vi "base.vi"() -> ()   [LabVIEW 2017]
uses:
  <vilib>/Analysis/baseanly.llb/Inverse f Filter (DBL).vi
  <vilib>/Analysis/NI_AALBase.lvlib
panel:
  out "LED":bool
  in  "stop 3":bool
  in  "Amplitude du signal":dbl(knob) scale=0.0..10.0
  out "Valeur pic à pic du signal":dbl
  out "Graphe 2":dynamicdata(graph)
  in  "Bouton rotatif":dbl(knob) scale=0.0..10.0
  in  "stop 2":bool
  out "Graphe":dynamicdata(graph)
  out "Tableau aléatoire de nombres compris entre 0 et 20":dbl[](array[numeric])
  in  "stop":bool
  out "u":dbl[](array[numeric])
  in  "u0":dbl
  in  "q":dbl
  out "LED":bool
  in  "a":bool
  in  "b":bool
  in  "Numérique":i32
  out "u(n)":dbl[](array[numeric])
  out "u(N)":dbl
  in  "N":dbl
  out "sqrt(z)":dbl
  in  "z":dbl
  out "x = y ?":bool
  out "x < y ?":bool
  out "x > y ?":bool
  in  "Y":dbl
  in  "X":dbl
  out "F":dbl(slide) scale=0.0..100.0
  in  "C":dbl(slide) scale=0.0..100.0
  out "c 4":dbl
  in  "b 4":dbl
  in  "a 4":dbl
  out "c 3":dbl
  in  "b 3":dbl
  in  "a 3":dbl
  out "c 2":dbl
  in  "b 2":dbl
  in  "a 2":dbl
  out "c":dbl
  in  "b":dbl
  in  "a":dbl
  # "+"
  # "-"
  # "x"
  # "/"
  # "°F = 1,8 x °C + 32"
  # "u(N) = 2N + 1"
  # "u(n) = 3n+4"
  # "a ET b"
  # "suite géométrique"
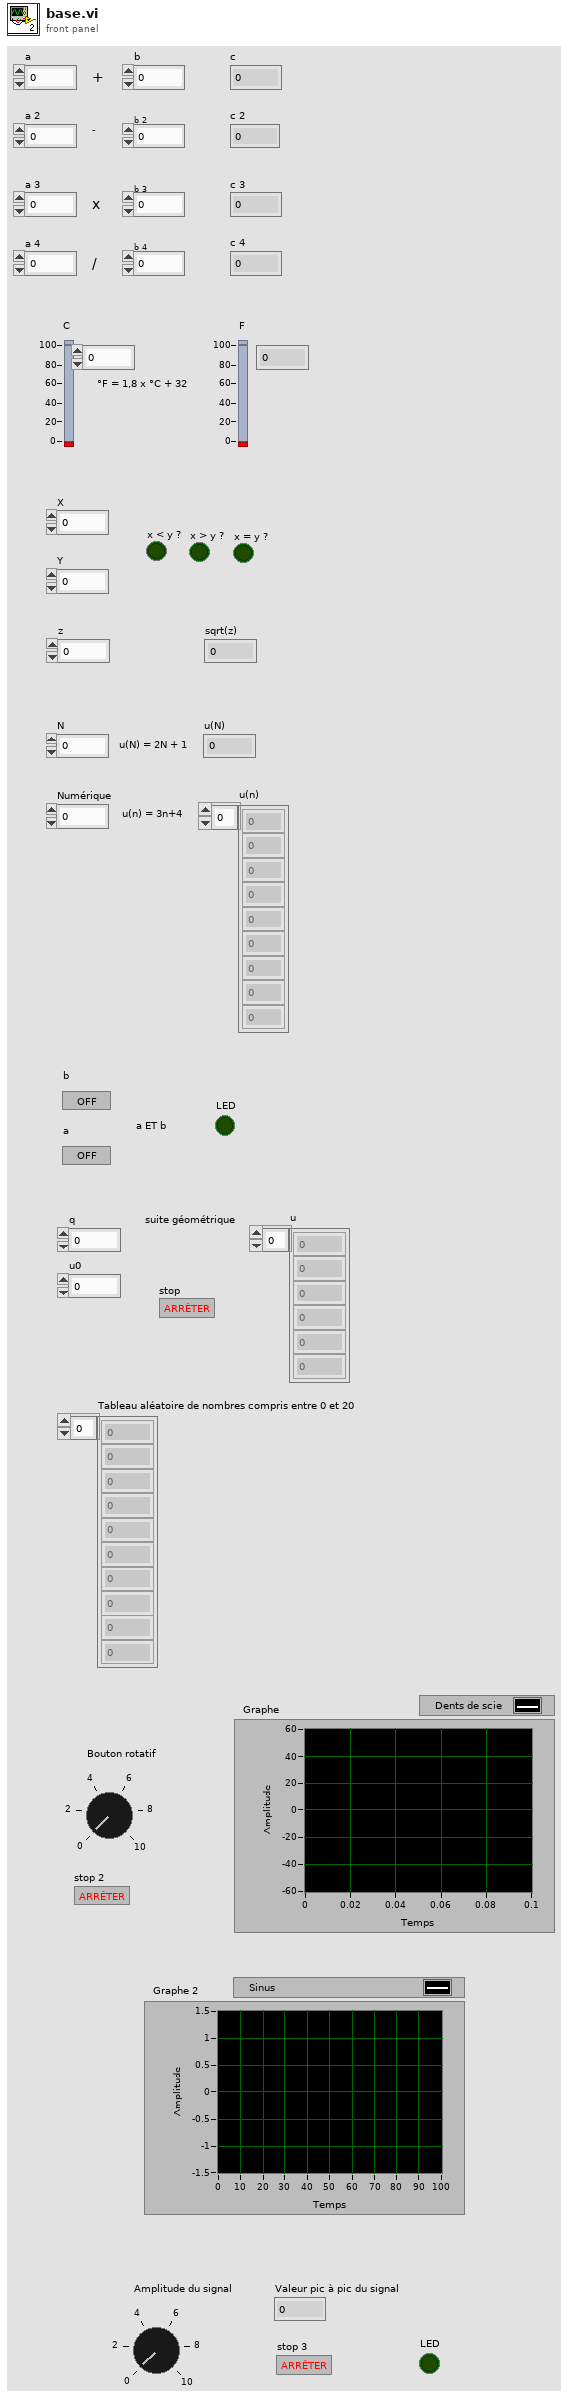
[diagram p1: front panel]
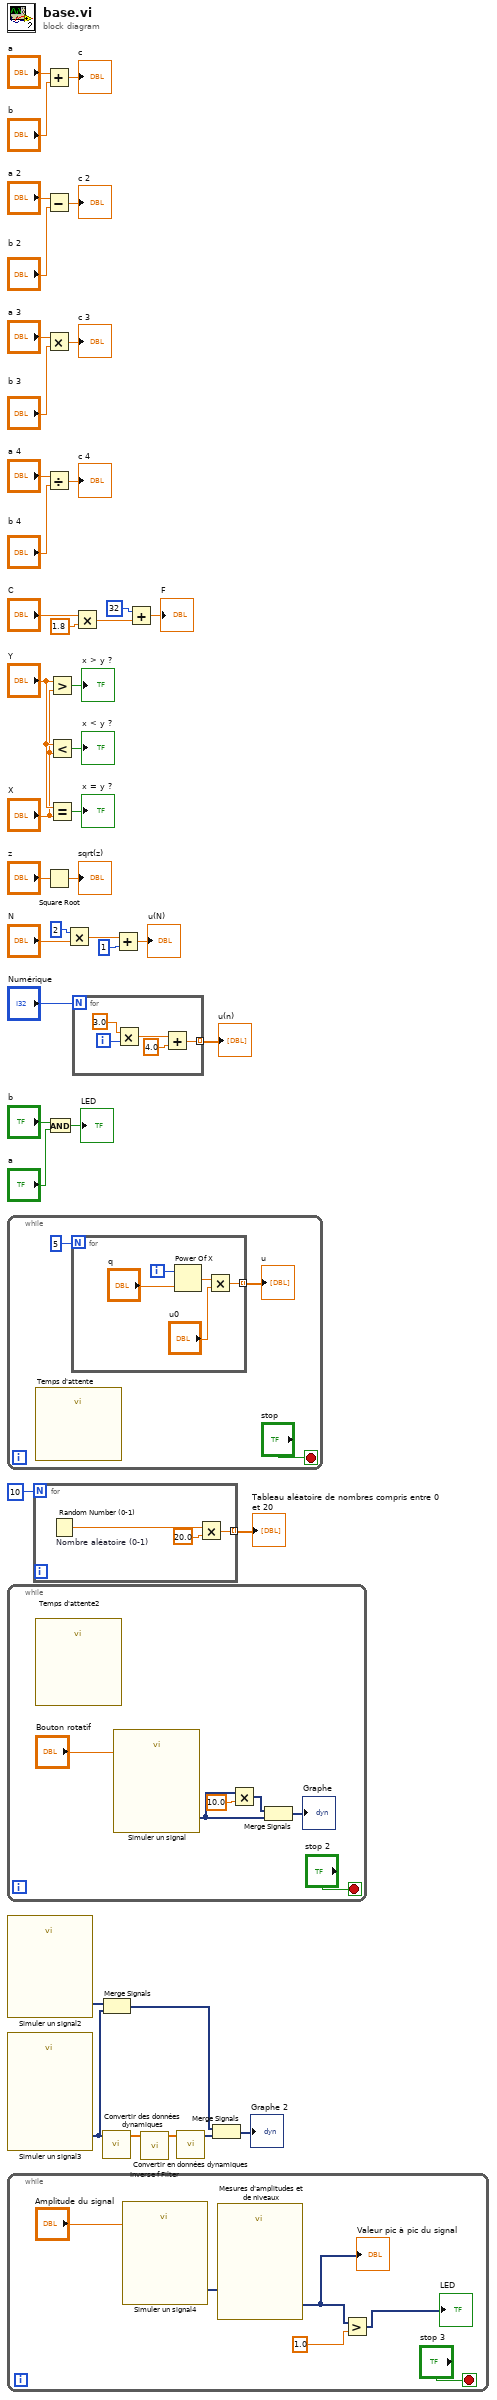
[diagram p0: block diagram]
diagram:
  n1 = while {
    stop <- "stop" stop-if-true
    n2 = call "Temps d'attente"() -> ()  [unwired: 11 in, 1 out]
    n3 = for {
      N: 5 -> [_]
      tunnel: [w48] -> w46 mode=indexing
      i -> [w47]
      n4 = Power Of X(1:"q", 2:w47) -> (0:w50:dbl)
      n5 = Multiply(x=w50, y="u0") -> (x*y=w48:dbl)
    }
    "u" <- w46
  }
  n6 = while {
    stop <- "stop 2" stop-if-true
    n7 = call "Temps d'attente2"() -> ()  [unwired: 11 in, 1 out]
    n8 = call "Simuler un signal"("Amplitude"="Bouton rotatif") -> ("Dents de scie"=w54:dynamicdata)  [unwired: 13 in, 1 out]
    n9 = Multiply(x=w54, y=10.0) -> (x*y=w57:dynamicdata)
    n10 = Merge Signals(w57, w54) -> (→"Graphe":dynamicdata)
  }
  n11 = call "Simuler un signal2"() -> ("Sinus"=w7:dynamicdata)  [unwired: 14 in, 1 out]
  n12 = call "Simuler un signal3"() -> ("Sinus avec Bruit uniforme"=w5:dynamicdata)  [unwired: 14 in, 1 out]
  n13 = while {
    stop <- "stop 3" stop-if-true
    n14 = call "Simuler un signal4"("Amplitude"="Amplitude du signal") -> ("Sinus"=w62:dynamicdata)  [unwired: 13 in, 1 out]
    n15 = call "Mesures d'amplitudes et de niveaux"("Signals"=w62) -> ("Peak to Peak"=w59:dynamicdata)  [unwired: 13 in, 1 out]
    "Valeur pic à pic du signal" <- w59
    n16 = Greater?(x=w59, y=1.0) -> (0:→"LED":dynamicdata)
  }
  n17 = for {
    N: 10 -> [_]
    tunnel: [w64] -> w8 mode=indexing
    n18 = Random Number (0-1) "Nombre aléatoire (0-1)"() -> (number: 0 to 1=w66:dbl)
    n19 = Multiply(x=w66, y=20.0 ("x*y")) -> (x*y=w64:dbl)
  }
  "Tableau aléatoire de nombres compris entre 0 et 20" <- w8
  n20 = Add(x="a", y="b") -> (x+y=→"c":dbl)
  n21 = Subtract(x="a 2", y="b 2") -> (x-y=→"c 2":dbl)
  n22 = Multiply(x="a 3", y="b 3") -> (x*y=→"c 3":dbl)
  n23 = Divide(x="a 4", y="b 4") -> (x/y=→"c 4":dbl)
  n24 = Square Root(x="z") -> (sqrt(x)=→"sqrt(z)":dbl)
  n25 = And(x="b", y="a") -> (x .and. y?=→"LED":bool)
  n26 = Greater?(x="Y", y="X") -> (0:→"x > y ?":bool)
  n27 = Less?(x="Y", y="X") -> (x < y?=→"x < y ?":bool)
  n28 = Equal?(x="Y", y="X") -> (x = y?=→"x = y ?":bool)
  n29 = Multiply(x=2, y="N") -> (x*y=w17:dbl)
  n30 = for {
    N: "Numérique" -> [_]
    tunnel: [w71] -> w14 mode=indexing
    i -> [w67]
    n31 = Multiply(x=3.0 ("y"), y=w67) -> (x*y=w70:dbl)
    n32 = Add(x=w70, y=4.0 ("x+y")) -> (x+y=w71:dbl)
  }
  "u(n)" <- w14
  n33 = Multiply(x="C", y=1.8) -> (x*y=w29:dbl)
  n34 = call "Convertir des données dynamiques"("Dynamic Data Type"=w5) -> ("Array"=w4:dbl[])  [unwired: 3 in]
  n35 = Merge Signals(w7, w5) -> (w6:dynamicdata)
  n36 = Add(x=w17, y=1) -> (x+y=→"u(N)":dbl)
  n37 = Add(x=32, y=w29) -> (x+y=→"F":dbl)
  n38 = call-poly <vilib>:"Inverse f Filter.vi"("X"=w4) -> ("Filtered X"=w2:dbl[])  [unwired: 6 in, 4 out]
  n39 = call "Convertir en données dynamiques"("Array"=w2) -> ("Dynamic Data Type"=w1:dynamicdata)  [unwired: 3 in]
  n40 = Merge Signals(w6, w1) -> (→"Graphe 2":dynamicdata)
